vi "Split.vi"(8 "Split Threshold":dbl=0.2, 11 "Original Line":T1={"Points"=[{"X"=0.0, "Y"=0.0}, {"X"=1.0, "Y"=1.0}, {"X"=2.0, "Y"=2.0}, {"X"=3.0, "Y"=3.0}, {"X"=4.0, "Y"=2.0}, {"X"=5.0, "Y"=1.0}, {"X"=6.0, "Y"=0.0}]}) -> (3 "Resulting Lines":T1[](array[typedef]))   [LabVIEW 2017]
uses:
  Vector Library/Line.ctl
  Vector Library/Vector.ctl
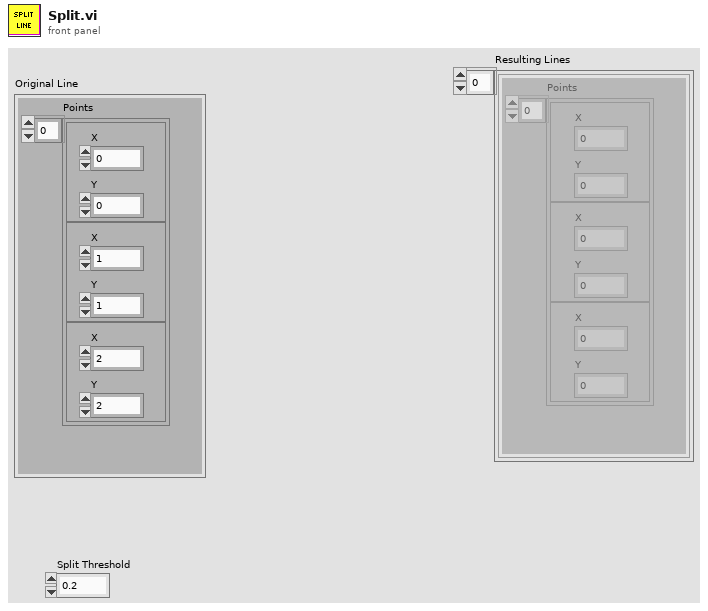
[diagram p1: front panel]
types:
  T1 = typedef "Line.ctl" = cluster{"Points":T2[]}
  T2 = typedef "Vector.ctl" = cluster{"X":dbl, "Y":dbl}
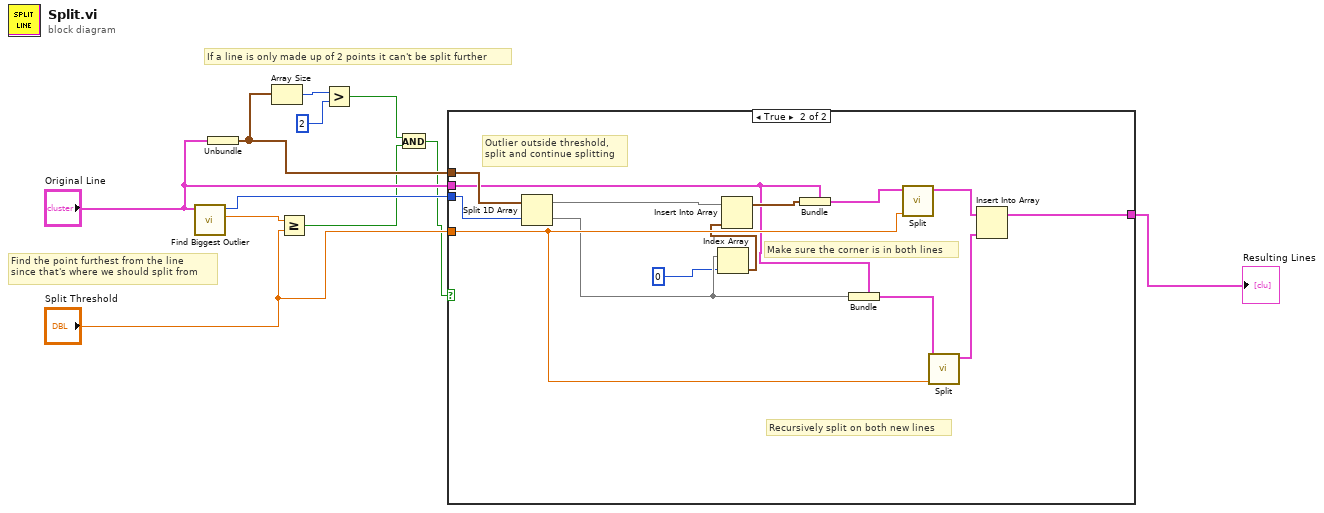
[diagram p0: block diagram]
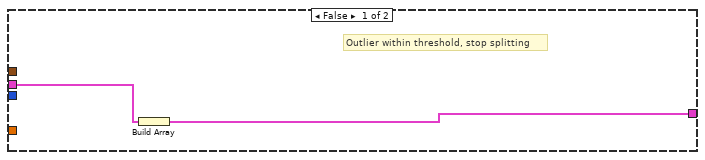
[diagram p2: hidden frame]
diagram:
  # "Find the point furthest from the line\nsince that's where we should split from"
  # "If a line is only made up of 2 points it can't be split further"
  n1 = call "Find Biggest Outlier.vi"("Line with outlier"="Original Line") -> ("Outlier Amount"=w9:dbl, "Outlier Index"=w8:i32)  [unwired: 9 in]
  n2 = Unbundle("Original Line") -> ("Points"=w7:T2[])
  n3 = Array Size(array=w7) -> (size(s)=w5:i32)
  n4 = Greater Or Equal?(x=w9, y="Split Threshold") -> (x >= y?=w3:bool)
  n5 = Greater?(x=w5, y=2) -> (0:w4:bool)
  n6 = And(x=w4, y=w3) -> (x .and. y?=w2:bool)
  n7 = case shown="False" w2 {
    tunnel: w8 -> [_ w20]
    tunnel: w7 -> [_ w27]
    tunnel: "Original Line" -> [w13 w14]
    tunnel: "Split Threshold" -> [_ w24]
    tunnel: [w12 w21] -> w1
    frame False {
      # "Outlier within threshold, stop splitting"
      n8 = Build Array(w13) -> (w12:T1[])
    }
    frame True {
      # "Recursively split on both new lines"
      # "Make sure the corner is in both lines"
      # "Outlier outside threshold,\nsplit and continue splitting"
      n9 = Split 1D Array(array=w27, index=w20) -> (first subarray=w18:T2[], second subarray=w19:T2[])
      n10 = Index Array(array=w19, index=0) -> (element=w15:T2)
      n11 = Insert Into Array(array=w18, new element=w15) -> (w17:T2[])  [unwired: 1 in]
      n12 = Bundle(cluster=w14, "Points"=w17) -> (w26:T1)
      n13 = Bundle(cluster=w14, "Points"=w19) -> (w25:T1)
      n14 = call "Split.vi"("Split Threshold"=w24, "Original Line"=w26) -> ("Resulting Lines"=w23:T1[])  [unwired: 9 in]
      n15 = call "Split.vi"("Split Threshold"=w24, "Original Line"=w25) -> ("Resulting Lines"=w22:T1[])  [unwired: 9 in]
      n16 = Insert Into Array(array=w23, new element=w22) -> (w21:T1[])  [unwired: 1 in]
    }
  }
  "Resulting Lines" <- w1
